vi "json_array.vi"(5 "text":string, 7 "ch":string, 9 "at":i32, 11 "error in (no error)":errorcluster) -> (4 "array":variant, 6 "text dup":string, 8 "ch out":string, 10 "at out":i32, 15 "error out":errorcluster)   [LabVIEW 2011]
doc: "Recursively generate an array. Mixed type arrays will be represented as a variant with attributes. Each element of the array will be named with its index: 0, 1, 2, etc. Single type arrays will also have an \"array\" attribute, containing an array of the correct type."
uses:
  <vilib>/Utility/VariantDataType/Type.ctl
  <vilib>/Utility/VariantDataType/VariantType.lvlib
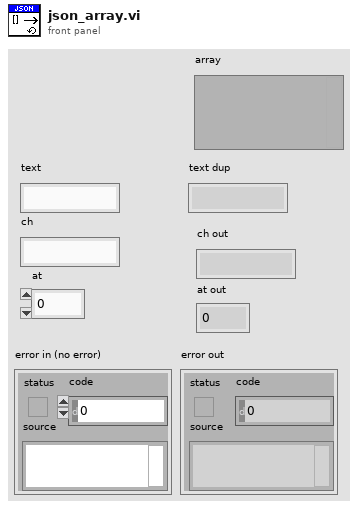
[diagram p1: front panel]
types:
  T1 = typedef "VariantType.lvlib/Type.ctl" = enum8{"Invalid Type", "Void", "I8", "I16", "I32", "I64", "U8", "U16", "U32", "U64", "Single Float", "Double Float", "Extended Float", "Single Complex", "Double Complex", "Extended Complex", "Enum U8", "Enum U16", "Enum U32", "Enum U64", "Single Float With Unit", "Double Float With Unit", "Extended Float With Unit", "Single Complex with Unit", "Double Complex with Unit", "Extended Complex with Unit", "Boolean", "String", "Path", "Picture", "Tag", "Array", "Cluster", "Variant", "LV Variant", "Waveform", "Timestamp", "Digital Waveform", "Digital Data", "ExpressData", "Refnum", "External Data", "VI", "Poly VI", "LabVIEW Class Instance", "Fixed Point"}
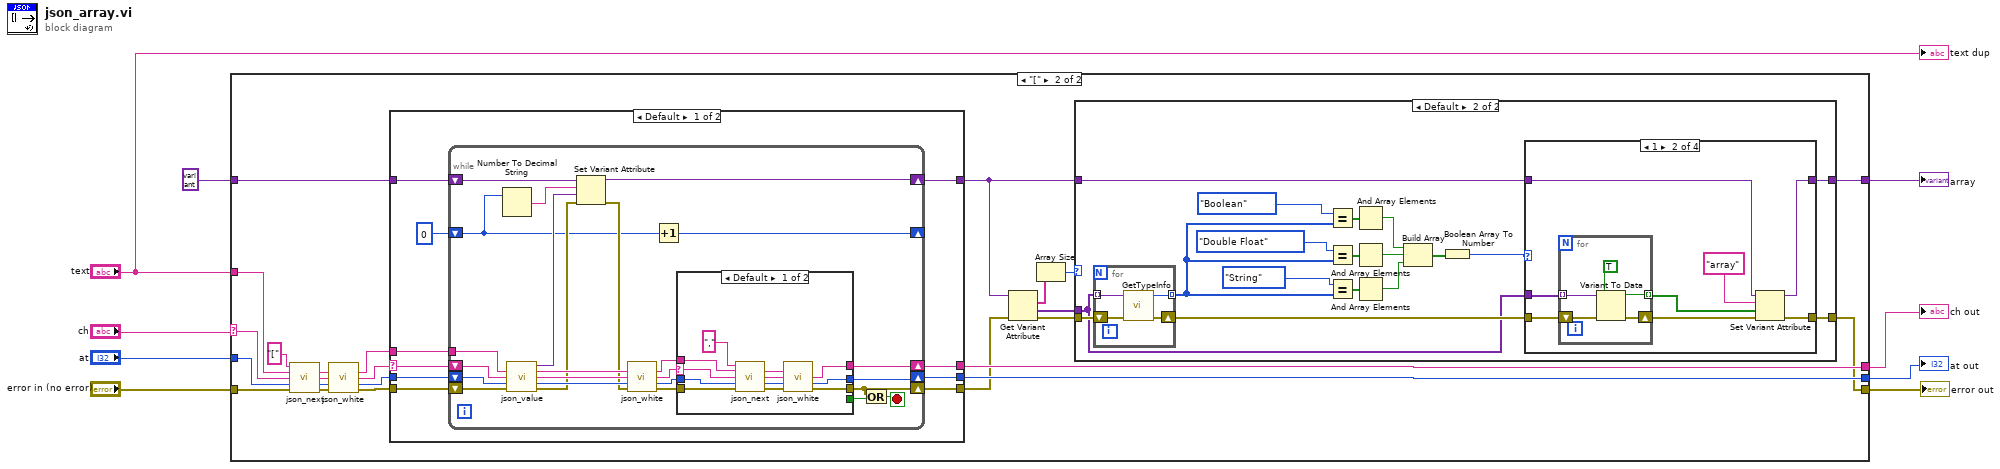
[diagram p0: block diagram]
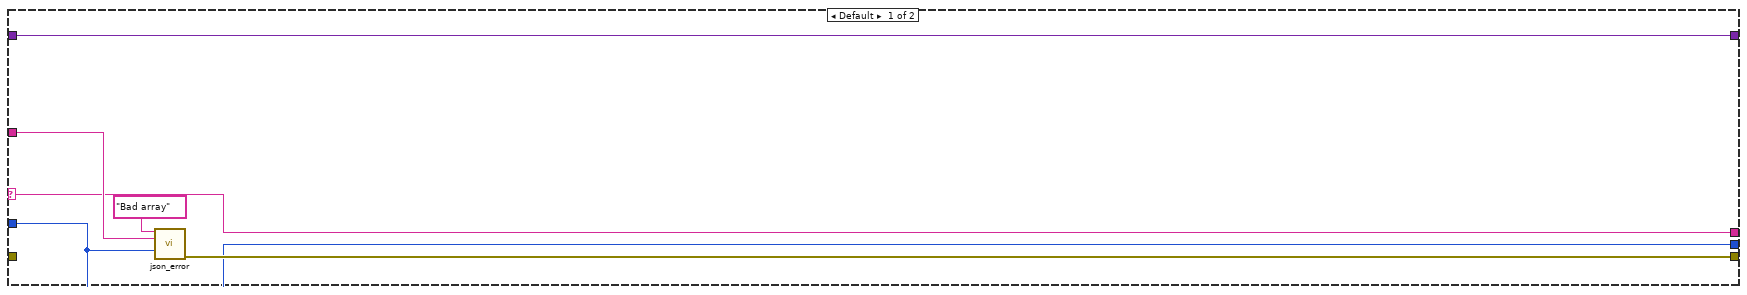
[diagram p2: hidden frame]
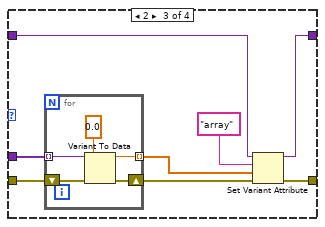
[diagram p5: hidden frame]
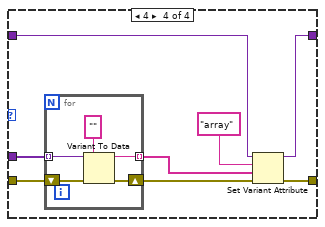
[diagram p6: hidden frame]
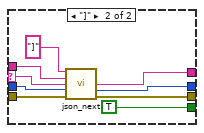
[diagram p7: hidden frame]
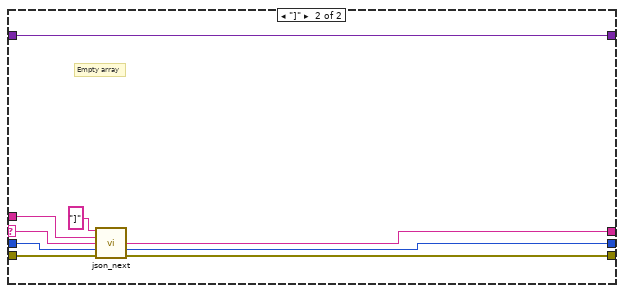
[diagram p8: hidden frame]
diagram:
  n1 = case shown="\"[\"" "ch" {
    selector: "ch" -> [w10 w37]
    tunnel: "error in (no error)" -> [_ w39]
    tunnel: [w13 w16] -> w8
    tunnel: variant ("array") -> [w12 w26]
    tunnel: "at" -> [w11 w38]
    tunnel: "text" -> [w15 w36]
    tunnel: [w12 w18] -> w3
    tunnel: [w11 w25] -> w2
    tunnel: [w10 w24] -> w1
    frame Default {
      n2 = call "json_error.vi"("m"="Bad array", "text"=w15, "at"=w11) -> ("error out"=w13:errorcluster)  [unwired: 12 in]
    }
    frame "[" {
      n3 = call "json_next.vi"("c"="[", "text"=w36, "ch"=w37, "at"=w38, "error in (no error)"=w39) -> ("text dup"=w31:string, "ch out"=w32:string, "at out"=w33:i32, "error out"=w34:errorcluster)  [unwired: 7 in]
      n4 = call "json_white.vi"("text"=w31, "ch"=w32, "at"=w33, "error in (no error)"=w34) -> ("text dup"=w27:string, "ch out"=w30:string, "at out"=w29:i32, "error out"=w28:errorcluster)  [unwired: 8 in]
      n5 = case shown="Default" w30 {
        selector: w30 -> [w112 w164]
        tunnel: w29 -> [w113 w165]
        tunnel: w28 -> [w114 w167]
        tunnel: w27 -> [w111 w163]
        tunnel: [w107 w166] -> w23
        tunnel: w26 -> [w109 w168]
        tunnel: [w108 w168] -> w19
        tunnel: [w106 w160] -> w25
        tunnel: [w105 w161] -> w24
        frame Default {
          n6 = while {
            shift-right: [w117] -> w107
            shift-left: w114 -> [w138]
            shift-right: [w128] -> w106
            shift-left: w113 -> [w137]
            shift-right: [w126] -> w105
            shift-left: w112 -> [w136]
            tunnel: w111 -> [w135]
            shift-right: [w118] -> _
            shift-left: 0 -> [w119]
            shift-right: [w120] -> w108
            shift-left: w109 -> [w125]
            stop <- w116 stop-if-true
            n7 = Number To Decimal String(number=w119) -> (decimal integer string=w124:string)  [unwired: 1 in]
            n8 = call "json_value.vi"("text"=w135, "ch"=w136, "at"=w137, "error in (no error)"=w138) -> ("value"=w123:variant, "text dup"=w133:string, "ch out"=w132:string, "at out"=w131:i32, "error out"=w122:errorcluster)  [unwired: 7 in]
            n9 = Set Variant Attribute(Variant=w125, name=w124, value=w123, error in=w122) -> (Variant out=w120:variant, error out=w121:errorcluster)  [unwired: 1 out]
            n10 = call "json_white.vi"("text"=w133, "ch"=w132, "at"=w131, "error in (no error)"=w121) -> ("text dup"=w127:string, "ch out"=w130:string, "at out"=w129:i32, "error out"=w134:errorcluster)  [unwired: 8 in]
            n11 = Increment(x=w119) -> (x+1=w118:i32)
            n12 = case shown="Default" w130 {
              selector: w130 -> [w148 w153]
              tunnel: w134 -> [w150 w158]
              tunnel: w129 -> [w149 w155]
              tunnel: [_ TRUE] -> w115
              tunnel: [w141 w157] -> w117
              tunnel: [w140 w156] -> w128
              tunnel: w127 -> [w147 w154]
              tunnel: [w139 w151] -> w126
              frame Default {
                n13 = call "json_next.vi"("c"=",", "text"=w147, "ch"=w148, "at"=w149, "error in (no error)"=w150) -> ("text dup"=w142:string, "ch out"=w143:string, "at out"=w144:i32, "error out"=w145:errorcluster)  [unwired: 7 in]
                n14 = call "json_white.vi"("text"=w142, "ch"=w143, "at"=w144, "error in (no error)"=w145) -> ("ch out"=w139:string, "at out"=w140:i32, "error out"=w141:errorcluster)  [unwired: 8 in, 1 out]
              }
              frame "]" {
                n15 = call "json_next.vi"("c"="]", "text"=w154, "ch"=w153, "at"=w155, "error in (no error)"=w158) -> ("ch out"=w151:string, "at out"=w156:i32, "error out"=w157:errorcluster)  [unwired: 7 in, 1 out]
              }
            }
            n16 = Or(x=w117, y=w115) -> (x .or. y?=w116:bool)
          }
        }
        frame "]" {
          # "Empty array"
          n17 = call "json_next.vi"("c"="]", "text"=w163, "ch"=w164, "at"=w165, "error in (no error)"=w167) -> ("ch out"=w161:string, "at out"=w160:i32, "error out"=w166:errorcluster)  [unwired: 7 in, 1 out]
        }
      }
      n18 = Get Variant Attribute(Variant=w19, error in=w23) -> (names=w21:string[], values=w22:variant[], error out=w17:errorcluster)  [unwired: 2 in, 1 out]
      n19 = Array Size(array=w21) -> (size(s)=w20:i32)
      n20 = case shown="Default" w20 {
        tunnel: w22 -> [_ w44]
        tunnel: w19 -> [w41 w55]
        tunnel: w17 -> [w40 w59]
        tunnel: [w41 w54] -> w18
        tunnel: [w40 w45] -> w16
        frame 0 {
        }
        frame Default {
          n21 = for {
            tunnel: w44 -> [w104] mode=indexing
            shift-right: [w102] -> w56
            shift-left: w59 -> [w103]
            tunnel: [w101] -> w51 mode=indexing
            n22 = call <vilib>:"GetTypeInfo.vi"("error in (no error)"=w103, "Variant"=w104) -> ("error out"=w102:errorcluster, "Type Enum"=w101:T1)  [unwired: 5 in, 3 out]
          }
          n23 = Equal?(x=Type."Boolean" ("Type Enum"), y=w51) -> (x = y?=w52:bool[])
          n24 = Equal?(x=Type."Double Float" ("Type Enum"), y=w51) -> (x = y?=w53:bool[])
          n25 = Equal?(x=Type."String" ("Type Enum"), y=w51) -> (x = y?=w57:bool[])
          n26 = And Array Elements(Boolean array=w52) -> (logical AND=w48:bool)
          n27 = And Array Elements(Boolean array=w53) -> (logical AND=w47:bool)
          n28 = And Array Elements(Boolean array=w57) -> (logical AND=w46:bool)
          n29 = Build Array(w48, w47, w46) -> (w43:bool[])
          n30 = Boolean Array To Number(Boolean array=w43) -> (number=w42:u32)
          n31 = case shown="1" w42 {
            tunnel: w56 -> [w60 w66 w79 w92]
            tunnel: w55 -> [w61 w68 w81 w94]
            tunnel: [w61 w67 w80 w93] -> w54
            tunnel: [w60 w69 w82 w95] -> w45
            tunnel: w44 -> [_ w65 w78 w91]
            frame Default {
              # "Mixed types,\ndon't add anything"
            }
            frame 1 {
              n32 = for {
                shift-right: [w73] -> w64
                shift-left: w66 -> [w74]
                tunnel: w65 -> [w72] mode=indexing
                tunnel: [w70] -> w63 mode=indexing
                n33 = Variant To Data(error in=w74, type=TRUE, Variant=w72) -> (data=w70:bool, error out=w73:errorcluster)
              }
              n34 = Set Variant Attribute(Variant=w68, name="array", value=w63, error in=w64) -> (Variant out=w67:variant, error out=w69:errorcluster)  [unwired: 1 out]
            }
            frame 2 {
              n35 = for {
                shift-right: [w86] -> w77
                shift-left: w79 -> [w87]
                tunnel: w78 -> [w85] mode=indexing
                tunnel: [w83] -> w76 mode=indexing
                n36 = Variant To Data(error in=w87, type=0.0, Variant=w85) -> (data=w83:dbl, error out=w86:errorcluster)
              }
              n37 = Set Variant Attribute(Variant=w81, name="array", value=w76, error in=w77) -> (Variant out=w80:variant, error out=w82:errorcluster)  [unwired: 1 out]
            }
            frame 4 {
              n38 = for {
                shift-right: [w99] -> w90
                shift-left: w92 -> [w100]
                tunnel: w91 -> [w98] mode=indexing
                tunnel: [w96] -> w89 mode=indexing
                n39 = Variant To Data(error in=w100, type="", Variant=w98) -> (data=w96:string, error out=w99:errorcluster)
              }
              n40 = Set Variant Attribute(Variant=w94, name="array", value=w89, error in=w90) -> (Variant out=w93:variant, error out=w95:errorcluster)  [unwired: 1 out]
            }
          }
        }
      }
    }
  }
  "error out" <- w8
  "array" <- w3
  "ch out" <- w1
  "at out" <- w2
  "text dup" <- "text"
